vi "Can Script Property Accessor.vi"(8 "error in (no error)":errorcluster, 11 "MultiDimArrElemScripter in":refnum<class "MultiDimArrElemScripter.lvclass">) -> (0 "error out":errorcluster, 2 "Can Script Property Accessor":bool, 3 "MultiDimArrElemScripter out":refnum<class "MultiDimArrElemScripter.lvclass">)   [LabVIEW 2021, in "MemberVICreation.lvlib" / "MultiDimArrElemScripter.lvclass"]
uses:
  <resource>/Framework/Providers/LVClassLibrary/NewAccessors/MultiDimArrElemScripter/MultiDimArrElemScripter.lvclass
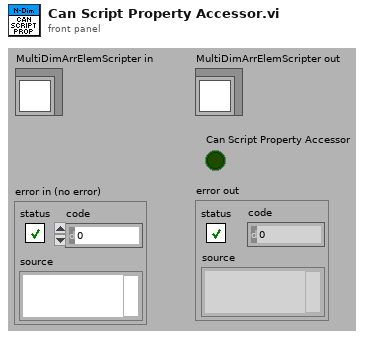
[diagram p1: front panel]
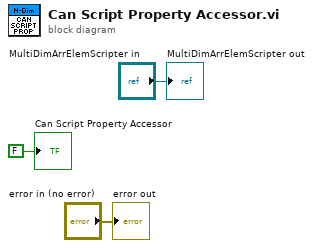
[diagram p0: block diagram]
diagram:
  "error out" <- "error in (no error)"
  "MultiDimArrElemScripter out" <- "MultiDimArrElemScripter in"
  "Can Script Property Accessor" <- FALSE ("Can Script Property Accessor")
